vi "OAT Overall Level Plot(XY) (N Channels).vi"(6 "X axis selection":u16(ring)=2 items=["Time", "Revolution", "RPM"], 7 "reset? (True)":bool=TRUE, 8 "speed profile":T1 {"speed [RPM]" format="%.2f"; "time [s]" format="%.2f"}, 9 "samples/rev":dbl=1.0 format="%.2f", 11 "overall level (even angular)":dbl[][](array[numeric]) format="%.2f") -> (1 "X unit":string, 3 "overall level":cluster{"X":dbl[], "Y":dbl[]}[](array[cluster]) {"Y" format="%.2f"; "X" format="%.2f"})   [LabVIEW 2017, in "SoundVib_Resampling.lvlib"]
uses:
  <vilib>/addons/Sound and Vibration/Order Analysis/Resample Order Tracking/SoundVib_Resampling.lvlib
  <vilib>/addons/Sound and Vibration/Order Analysis/Tach Process/SubVIs/speed profile.ctl
  <vilib>/Analysis/1siggen.llb/Ramp Pattern by Samples.vi
  <vilib>/Analysis/NI_AALBase.lvlib
  <vilib>/addons/Sound and Vibration/Order Analysis/Tach Process/SoundVib_TachProcess.lvlib
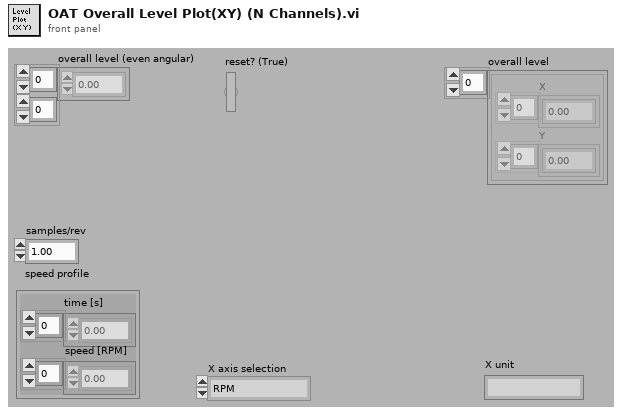
[diagram p1: front panel]
types:
  T1 = typedef "SoundVib_TachProcess.lvlib/speed profile.ctl" = cluster{"time [s]":dbl[], "speed [RPM]":dbl[]}
  T2 = cluster{"speed [RPM]":dbl[], "overall level (even angular)":dbl[]}
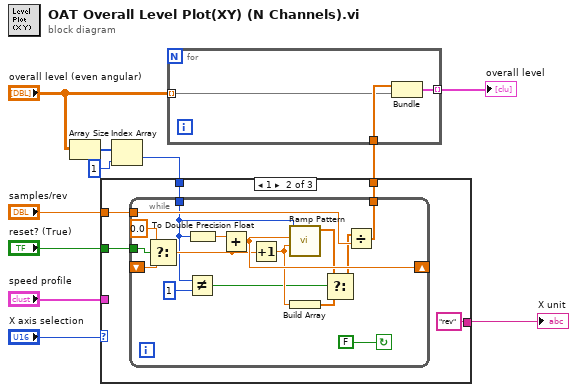
[diagram p0: block diagram]
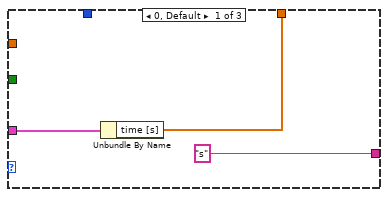
[diagram p2: hidden frame]
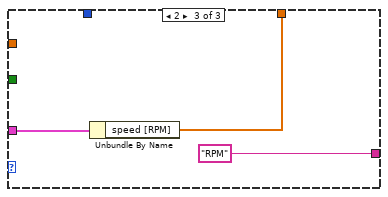
[diagram p3: hidden frame]
diagram:
  n1 = Array Size(array="overall level (even angular)") -> (size(s)=w9:i32[])
  n2 = Index Array(array=w9, index=1) -> (element=w6:i32)
  n3 = case shown="1" "X axis selection" {
    tunnel: "speed profile" -> [w14 _ w38]
    tunnel: [w13 w19 w37] -> w7
    tunnel: w6 -> [_ w15 _]
    tunnel: "samples/rev" -> [_ w17 _]
    tunnel: ["s" "rev" "RPM"] -> w3
    tunnel: "reset? (True)" -> [_ w16 _]
    frame 0, Default {
      n4 = Unbundle By Name(w14) -> ("time [s]"=w13:dbl[])
    }
    frame 1 {
      n5 = while {
        tunnel: [w35] -> w19
        tunnel: w17 -> [w34]
        tunnel: w16 -> [w32]
        shift-right: [w29] -> _
        shift-left: _ -> [w30]
        tunnel: w15 -> [w26]
        stop <- FALSE continue-if-true
        n6 = Select(t=0.0 ("f"), s=w32, f=w30) -> (s? t:f=w28:dbl)
        n7 = Not Equal?(x=w26, y=1) -> (x != y?=w24:bool)
        n8 = To Double Precision Float(number=w26) -> (double precision float=w20:dbl)
        n9 = Add(x=w20, y=w28) -> (x+y=w29:dbl)
        n10 = Increment(x=w28) -> (x+1=w25:dbl)
        n11 = call-poly <vilib>:"Ramp Pattern.vi"("start"=w25, "end"=w29, "samples"=w26) -> ("Ramp Pattern"=w23:dbl[])  [unwired: 7 in, 1 out]
        n12 = Build Array(w25) -> (w22:dbl[])
        n13 = Select(t=w23, s=w24, f=w22) -> (s? t:f=w21:dbl[])
        n14 = Divide(x=w21, y=w34) -> (x/y=w35:dbl[])
      }
    }
    frame 2 {
      n15 = Unbundle By Name(w38) -> ("speed [RPM]"=w37:dbl[])
    }
  }
  "X unit" <- w3
  n16 = for {
    tunnel: [w41] -> w4 mode=indexing
    tunnel: "overall level (even angular)" -> [w39] mode=indexing
    tunnel: w7 -> [w40]
    n17 = Bundle("speed [RPM]"=w40, "overall level (even angular)"=w39) -> (w41:T2)  [unwired: 1 in]
  }
  "overall level" <- w4
